vi "Rotating joystick by fixed angle.vi"() -> ()   [LabVIEW 2012]
panel:
  out "Y axis out":dbl
  out "X axis out":dbl
  in  "Rotate by angle":dbl
  in  "Y axis in":dbl
  in  "X axis in":dbl
  # "Clock wise"
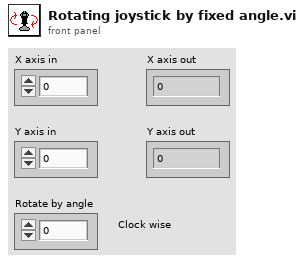
[diagram p1: front panel]
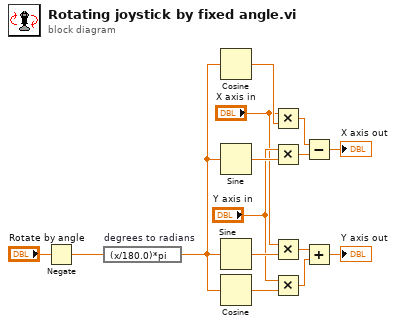
[diagram p0: block diagram]
diagram:
  n1 = Negate(x="Rotate by angle") -> (-x=w1:dbl)
  n2 = expression code="(x/180.0)*pi" "degrees to radians"(w1) -> (w6:dbl)
  n3 = Cosine(x=w6) -> (cos(x)=w14:dbl)
  n4 = Sine(x=w6) -> (sin(x)=w11:dbl)
  n5 = Sine(x=w6) -> (sin(x)=w5:dbl)
  n6 = Cosine(x=w6) -> (cos(x)=w4:dbl)
  n7 = Multiply(x="X axis in", y=w14) -> (x*y=w13:dbl)
  n8 = Multiply(x="Y axis in", y=w11) -> (x*y=w12:dbl)
  n9 = Multiply(x="X axis in", y=w5) -> (x*y=w9:dbl)
  n10 = Multiply(x="Y axis in", y=w4) -> (x*y=w8:dbl)
  n11 = Subtract(x=w13, y=w12) -> (x-y=→"X axis out":dbl)
  n12 = Add(x=w9, y=w8) -> (x+y=→"Y axis out":dbl)
